vi "t16subvi.vi"(10 "Método":enum16{"G", "Gx", "Gy"}(ring), 11 "Ruta":path) -> (3 "2D Picture":picture)   [LabVIEW 2020]
panel:
  # "Ceballos Conde Emanuel\n4MV6\nSistemas de visión artificial\n2022/1"
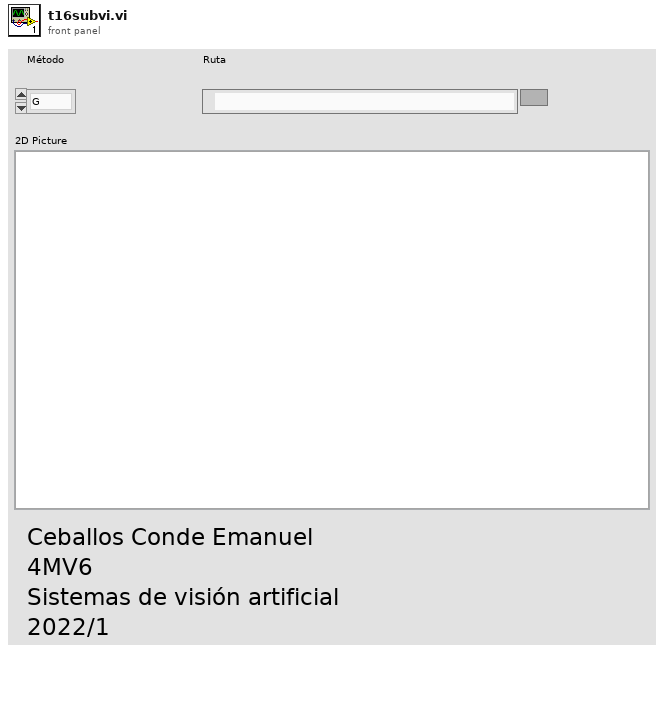
[diagram p1: front panel]
types:
  T1 = typedef "imagedata.ctl" = cluster{"image type":i32, "image depth":i32, "image":u8[], "mask":u8[], "colors":u32[], "Rectangle":cluster{"left":i16, "top":i16, "right":i16, "bottom":i16}}
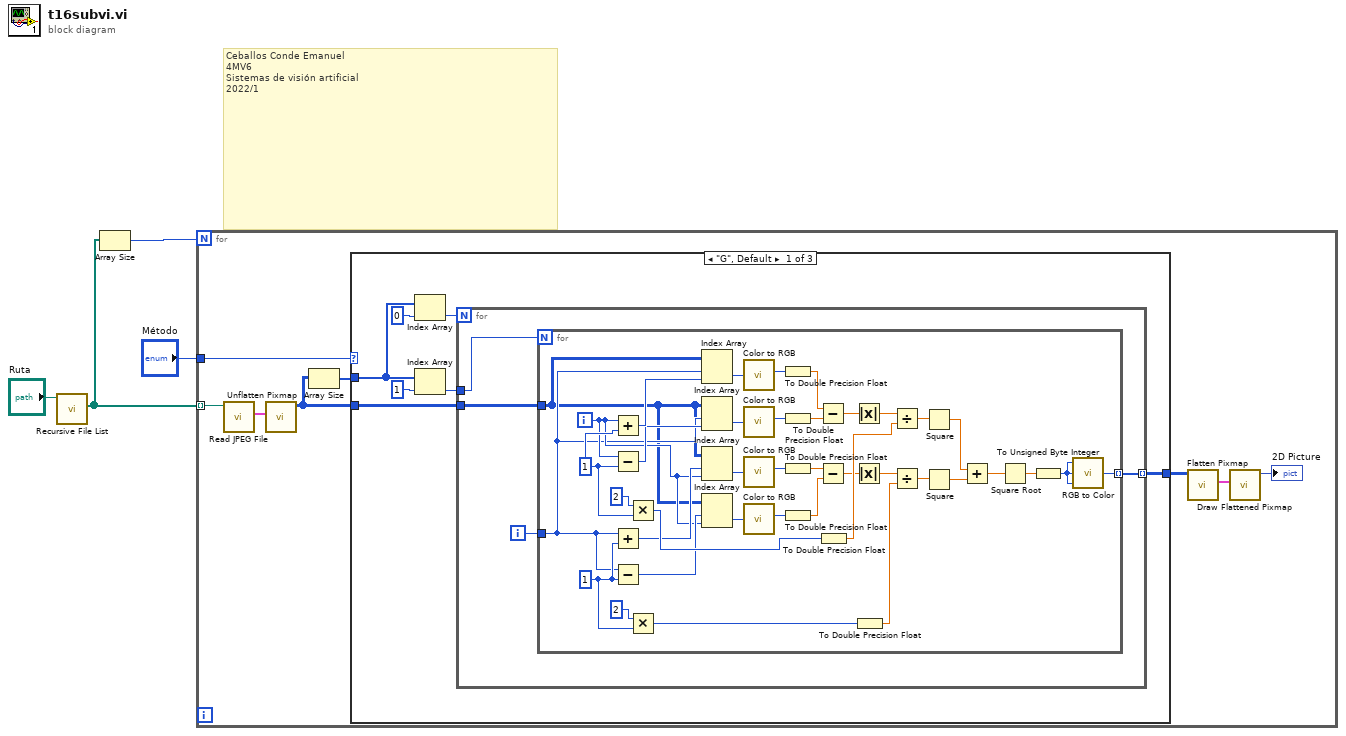
[diagram p0: block diagram]
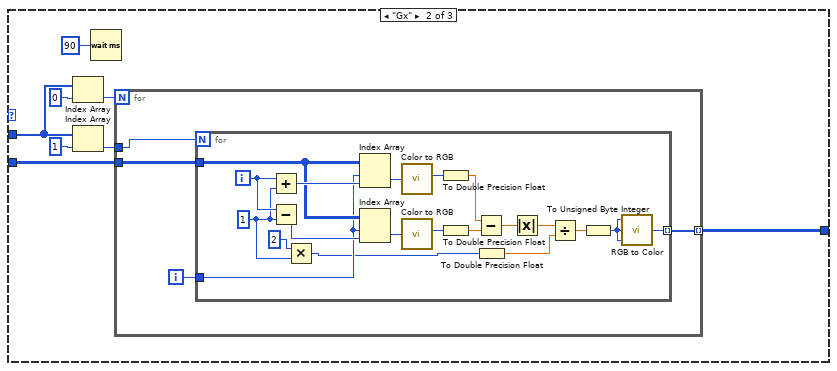
[diagram p2: hidden frame]
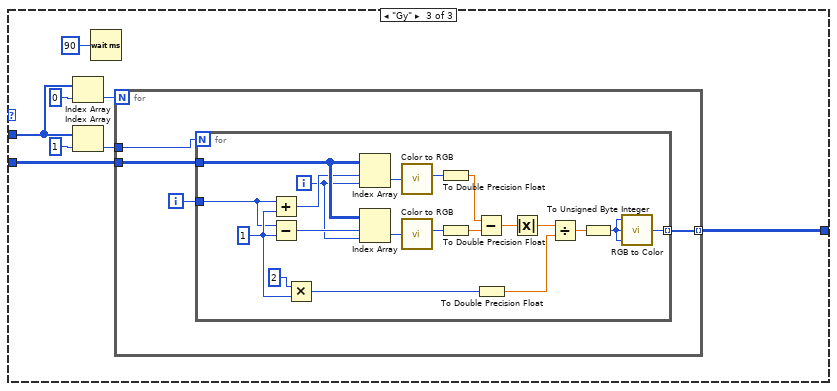
[diagram p3: hidden frame]
diagram:
  # "Ceballos Conde Emanuel\n4MV6\nSistemas de visión artificial\n2022/1"
  n1 = call <vilib>:"Recursive File List.vi"("Folder Path"="Ruta") -> ("All Files in Dir"=w4:path[])  [unwired: 6 in, 4 out]
  n2 = Array Size(array=w4) -> (size(s)=w3:i32)
  n3 = for {
    N: w3 -> [_]
    tunnel: w4 -> [w9] mode=indexing
    tunnel: "Método" -> [w5]
    n4 = call <vilib>:"Read JPEG File.vi"("path to JPEG file"=w9) -> ("image data"=w12:T1)  [unwired: 8 in, 2 out]
    n5 = call <vilib>:"Unflatten Pixmap.vi"("image data"=w12) -> ("24-bit pixmap"=w11:u32[][])  [unwired: 4 in, 6 out]
    n6 = Array Size(array=w11) -> (size(s)=w10:i32[])
    n7 = case shown="\"G\", Default" w5 {
      tunnel: w11 -> [w14 w69 w97]
      tunnel: [w15 w70 w98] -> w6
      tunnel: w10 -> [w13 w65 w96]
      frame "G", Default {
        n8 = Index Array(array=w13, index=0) -> (element=w19:i32)
        n9 = Index Array(array=w13, index=1) -> (element=w17:i32)
        n10 = for {
          N: w19 -> [_]
          tunnel: w14 -> [w23]
          tunnel: [w21] -> w15 mode=indexing
          tunnel: w17 -> [w20]
          i -> [w22]
          n11 = for {
            N: w20 -> [_]
            tunnel: w23 -> [w30]
            tunnel: w22 -> [w31]
            tunnel: [w58] -> w21 mode=indexing
            i -> [w32]
            w40 = 1
            w53 = 1
            n12 = Add(x=w32, y=w53) -> (x+y=w60:i32)
            n13 = Subtract(x=w32, y=w53) -> (x-y=w59:i32)
            n14 = Add(x=w31, y=w40) -> (x+y=w34:i32)
            n15 = Subtract(x=w31, y=w40) -> (x-y=w33:i32)
            n16 = Multiply(x=2, y=w53) -> (x*y=w54:i32)
            n17 = Multiply(x=2, y=w40) -> (x*y=w41:i32)
            n18 = Index Array(array=w30, index (row)=w31, index (col)=w60) -> (element=w62:u32)
            n19 = Index Array(array=w30, index (row)=w31, index (col)=w59) -> (element=w61:u32)
            n20 = Index Array(array=w30, index (row)=w34, index (col)=w32) -> (element=w46:u32)
            n21 = Index Array(array=w30, index (row)=w33, index (col)=w32) -> (element=w45:u32)
            n22 = call <vilib>:"Color to RGB.vi"("Color"=w62) -> ("R"=w57:u8)  [unwired: 3 out]
            n23 = call <vilib>:"Color to RGB.vi"("Color"=w61) -> ("R"=w56:u8)  [unwired: 3 out]
            n24 = call <vilib>:"Color to RGB.vi"("Color"=w46) -> ("R"=w44:u8)  [unwired: 3 out]
            n25 = call <vilib>:"Color to RGB.vi"("Color"=w45) -> ("R"=w43:u8)  [unwired: 3 out]
            n26 = To Double Precision Float(number=w57) -> (double precision float=w50:dbl)
            n27 = To Double Precision Float(number=w56) -> (double precision float=w49:dbl)
            n28 = To Double Precision Float(number=w44) -> (double precision float=w37:dbl)
            n29 = To Double Precision Float(number=w43) -> (double precision float=w36:dbl)
            n30 = Subtract(x=w50, y=w49) -> (x-y=w55:dbl)
            n31 = Subtract(x=w37, y=w36) -> (x-y=w42:dbl)
            n32 = To Double Precision Float(number=w54) -> (double precision float=w48:dbl)
            n33 = Absolute Value(x=w55) -> (abs(x)=w51:dbl)
            n34 = Absolute Value(x=w42) -> (abs(x)=w38:dbl)
            n35 = To Double Precision Float(number=w41) -> (double precision float=w35:dbl)
            n36 = Divide(x=w51, y=w48) -> (x/y=w29:dbl)
            n37 = Divide(x=w38, y=w35) -> (x/y=w28:dbl)
            n38 = Square(x=w29) -> (x^2=w27:dbl)
            n39 = Square(x=w28) -> (x^2=w26:dbl)
            n40 = Add(x=w27, y=w26) -> (x+y=w25:dbl)
            n41 = Square Root(x=w25) -> (sqrt(x)=w24:dbl)
            n42 = To Unsigned Byte Integer(number=w24) -> (unsigned 8bit integer=w47:u8)
            n43 = call <vilib>:"RGB to Color.vi"("B"=w47, "G"=w47, "R"=w47) -> ("Color"=w58:u32)
          }
        }
      }
      frame "Gx" {
        n44 = Index Array(array=w65, index=0) -> (element=w68:i32)
        n45 = Index Array(array=w65, index=1) -> (element=w66:i32)
        n46 = Wait (ms)(milliseconds to wait=u32 90) -> ()  [unwired: 1 out]
        n47 = for {
          N: w68 -> [_]
          tunnel: w69 -> [w74]
          tunnel: [w72] -> w70 mode=indexing
          tunnel: w66 -> [w71]
          i -> [w73]
          n48 = for {
            N: w71 -> [_]
            tunnel: w74 -> [w89]
            tunnel: w73 -> [w88]
            tunnel: [w90] -> w72 mode=indexing
            i -> [w87]
            w82 = 1
            n49 = Add(x=w87, y=w82) -> (x+y=w92:i32)
            n50 = Subtract(x=w87, y=w82) -> (x-y=w91:i32)
            n51 = Multiply(x=2, y=w82) -> (x*y=w83:i32)
            n52 = Index Array(array=w89, index (row)=w88, index (col)=w92) -> (element=w94:u32)
            n53 = Index Array(array=w89, index (row)=w88, index (col)=w91) -> (element=w93:u32)
            n54 = call <vilib>:"Color to RGB.vi"("Color"=w94) -> ("R"=w86:u8)  [unwired: 3 out]
            n55 = call <vilib>:"Color to RGB.vi"("Color"=w93) -> ("R"=w85:u8)  [unwired: 3 out]
            n56 = To Double Precision Float(number=w86) -> (double precision float=w78:dbl)
            n57 = To Double Precision Float(number=w85) -> (double precision float=w77:dbl)
            n58 = Subtract(x=w78, y=w77) -> (x-y=w84:dbl)
            n59 = To Double Precision Float(number=w83) -> (double precision float=w76:dbl)
            n60 = Absolute Value(x=w84) -> (abs(x)=w79:dbl)
            n61 = Divide(x=w79, y=w76) -> (x/y=w80:dbl)
            n62 = To Unsigned Byte Integer(number=w80) -> (unsigned 8bit integer=w75:u8)
            n63 = call <vilib>:"RGB to Color.vi"("B"=w75, "G"=w75, "R"=w75) -> ("Color"=w90:u32)
          }
        }
      }
      frame "Gy" {
        n64 = Index Array(array=w96, index=0) -> (element=w101:i32)
        n65 = Index Array(array=w96, index=1) -> (element=w102:i32)
        n66 = Wait (ms)(milliseconds to wait=u32 90) -> ()  [unwired: 1 out]
        n67 = for {
          N: w101 -> [_]
          tunnel: w97 -> [w106]
          tunnel: [w104] -> w98 mode=indexing
          tunnel: w102 -> [w103]
          i -> [w105]
          n68 = for {
            N: w103 -> [_]
            tunnel: w106 -> [w123]
            tunnel: w105 -> [w108]
            tunnel: [w124] -> w104 mode=indexing
            i -> [w107]
            w118 = 1
            n69 = Add(x=w108, y=w118) -> (x+y=w110:i32)
            n70 = Subtract(x=w108, y=w118) -> (x-y=w109:i32)
            n71 = Multiply(x=2, y=w118) -> (x*y=w119:i32)
            n72 = Index Array(array=w123, index (row)=w110, index (col)=w107) -> (element=w126:u32)
            n73 = Index Array(array=w123, index (row)=w109, index (col)=w107) -> (element=w125:u32)
            n74 = call <vilib>:"Color to RGB.vi"("Color"=w126) -> ("R"=w122:u8)  [unwired: 3 out]
            n75 = call <vilib>:"Color to RGB.vi"("Color"=w125) -> ("R"=w121:u8)  [unwired: 3 out]
            n76 = To Double Precision Float(number=w122) -> (double precision float=w114:dbl)
            n77 = To Double Precision Float(number=w121) -> (double precision float=w113:dbl)
            n78 = Subtract(x=w114, y=w113) -> (x-y=w120:dbl)
            n79 = To Double Precision Float(number=w119) -> (double precision float=w112:dbl)
            n80 = Absolute Value(x=w120) -> (abs(x)=w115:dbl)
            n81 = Divide(x=w115, y=w112) -> (x/y=w116:dbl)
            n82 = To Unsigned Byte Integer(number=w116) -> (unsigned 8bit integer=w111:u8)
            n83 = call <vilib>:"RGB to Color.vi"("B"=w111, "G"=w111, "R"=w111) -> ("Color"=w124:u32)
          }
        }
      }
    }
    n84 = call <vilib>:"Flatten Pixmap.vi"("24-bit pixmap"=w6) -> ("image data"=w7:T1)  [unwired: 10 in]
    n85 = call <vilib>:"Draw Flattened Pixmap.vi"("image data"=w7) -> ("new picture"=→"2D Picture":picture)  [unwired: 8 in]
  }
